vi "Heat fuse RV1.vi"(8 "error in":errorcluster) -> (0 "error out":errorcluster, 1 "PASS/FAIL":bool, 2 "VHeatFuse_load":string, 3 "VHeatFuse_noload":string)   [LabVIEW 2009]
uses:
  Digit IO PCI 6503/Digit IO control.ctl
  Global/Global 1.vi
panel:
  out "status":bool
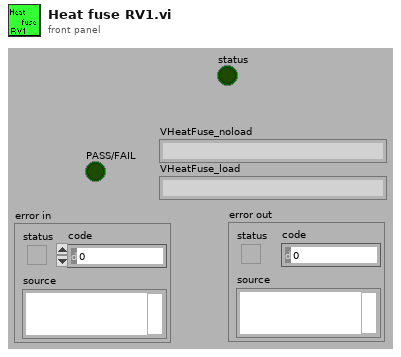
[diagram p1: front panel]
types:
  T1 = typedef "Digit IO control.ctl" = enum16{"Pull X1_4 Low", "Disconnect Pull X1_4 Low", "Down Cylinder", "Disconnect Down Cylinder", "Load X1_1_5", "Disconnect Load X1_1_5", "Measu X1_1_5", "Disconnect Measu X1_1_5", "Measu Z1_1_5", "Disconnect Measu Z1_1_5", "Power X1_1", "Disconnect Power X1_1", "RS232 Power", "Disconnect RS232 Power", "Card Cylinder", "Disconnect Card Cylinder", "Fail LED", "Disconnect Fail LED", "LCA Power", "Disconnect LCA Power", "BeyondCylinderDowndigit", "Disconnect BeyondCylinderDowendigit", "Frequency", "Disconnect Frequency", "Measu Current", "Disconnect Measu Current", "Measu current_1", "Disconnect Measu current_1", "Digit ALL", "Disconnect Digit ALL", "PASS LED", "Disconnect PASS LED", "Load Z1_1_3", "Disconnect Load Z1_1_3", "RS232 Connect", "Disconnect RS232 Connect", "Power Z1_7", "Disconnect Power Z1_7", "Pull Z_1_5  low", "Disconnect Pull Z_1_5  low", "Connect LCA_1", "Disconnect LCA_1", "short LCA", "Disconnect short LCA", "PT100", "Disconnect PT100", "NO connect", "Disconnect NO connect"}
  T2 = cluster{"VHEATFUSENOLOADMIN":string, "VHEATFUSELOADMAX":string, "VOVERRIDEDIODEMIN":string, "TDIFFMAX":string, "MEASFREQMAX":string, "MEASFREQMIN":string, "VOVER":string, "VMIDDLE":string, "VUNDER":string, "VNORESET":string, "VRESET":string, "WAITPING":string, "LRFID":string, "RFIDUID":string, "EXTEESIZE":string, "LCUTYPE":string, "LCUSUBTYPE":string, "TEVN":string, "BOOTVER":string, "APPVER":string, "ISLEEPMAX":string, "TSLEEP":string, "APPWAIT":string, "DBWAIT":string}
  T3 = cluster{"People":string, "product  number":string, "Test time":string, "VHeatFuse_noload":string, "VHeatFuse_load":string, "VoverrideDiode":string, "Test firmware upload via X1":string, "TemperAddress":string, "Troom":string, "TLCU":string, "Adjustment factor":string, "MeasuredFreq":string, "I2C communication":string, "Light-emitting diode on Z2":string, "Battery warning/inhibit":string, "Reset by IC10":string, "External EEPROM":string, "RFID card detection and reading RFID":string, "Production parameters in internal EEPROM":string, "Current consumption in sleep mode":string, "Application and database upload":string, "Test result":string, "Table head[22]":string, "Table head[23]":string}
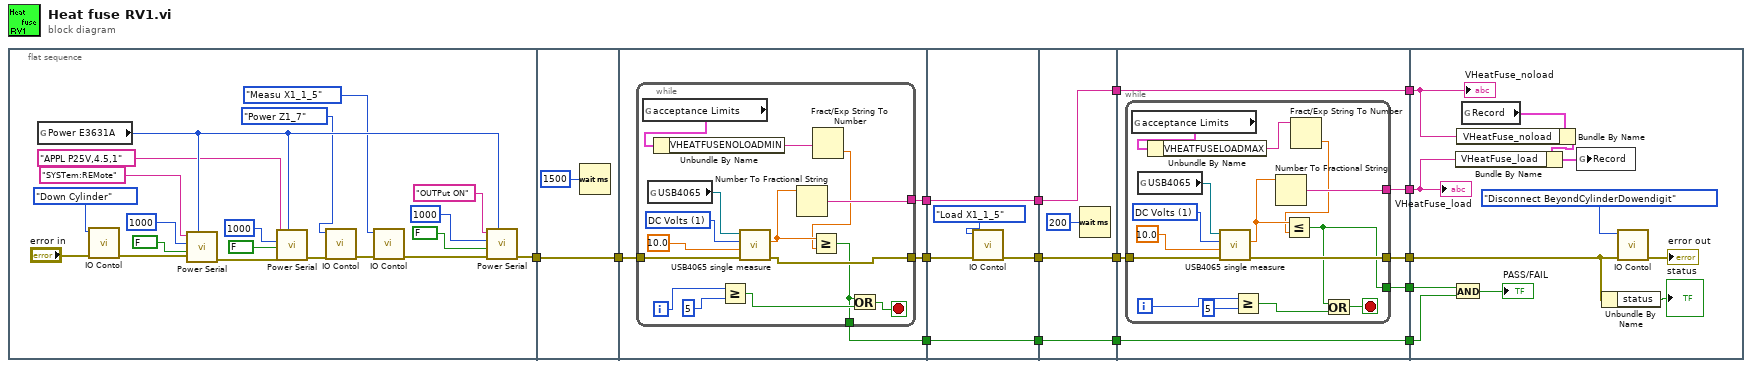
[diagram p0: block diagram]
diagram:
  n1 = flat-sequence {
    tunnel: [w33] -> w2
    tunnel: w2 -> [w37]
    tunnel: [w37] -> w1
    tunnel: [w42] -> w16
    tunnel: [w41] -> w8
    tunnel: [w40] -> w4
    tunnel: w1 -> [w39]
    tunnel: w16 -> [w62]
    tunnel: [w61] -> w14
    tunnel: [w59] -> w9
    tunnel: w8 -> [w59]
    tunnel: [w58] -> w5
    tunnel: w4 -> [w58]
    tunnel: [w65] -> w15
    tunnel: w14 -> [w65]
    tunnel: [w64] -> w10
    tunnel: w9 -> [w64]
    tunnel: [w63] -> w6
    tunnel: w5 -> [w63]
    tunnel: w15 -> [w72]
    tunnel: [w71] -> w13
    tunnel: [w70] -> w12
    tunnel: [w69] -> w11
    tunnel: w10 -> [w69]
    tunnel: [w68] -> w7
    tunnel: w6 -> [w68]
    tunnel: [w67] -> w3
    tunnel: w13 -> [w95]
    tunnel: w12 -> [w88]
    tunnel: w11 -> [w94]
    tunnel: w7 -> [w93]
    tunnel: w3 -> [w92]
    frame #0 {
      n2 = global read "Global 1.vi" "Power E3631A"() -> (w32:i32)
      n3 = call "IO Contol.vi"("error in"="error in", "IO Operation"=Digit_IO_control."Down Cylinder" ("Enum")) -> ("error out"=w17:errorcluster)  [unwired: 9 out]
      n4 = call "Power Serial.vi"("VISA Resource Address"=w32, "error in (no error)"=w17, "Rd?"=FALSE ("write"), "Delay"=1000, "IN"="SYSTem:REMote" ("In")) -> ("error out"=w24:errorcluster)  [unwired: 6 out]
      n5 = call "Power Serial.vi"("VISA Resource Address"=w32, "error in (no error)"=w24, "Rd?"=FALSE, "Delay"=1000, "IN"="APPL P25V,4.5,1" ("In")) -> ("error out"=w20:errorcluster)  [unwired: 6 out]
      n6 = call "IO Contol.vi"("error in"=w20, "IO Operation"=Digit_IO_control."Power Z1_7" ("Enum")) -> ("error out"=w30:errorcluster)  [unwired: 9 out]
      n7 = call "IO Contol.vi"("error in"=w30, "IO Operation"=Digit_IO_control."Measu X1_1_5" ("Enum")) -> ("error out"=w31:errorcluster)  [unwired: 9 out]
      n8 = call "Power Serial.vi"("VISA Resource Address"=w32, "error in (no error)"=w31, "Rd?"=FALSE, "Delay"=1000, "IN"="OUTPut ON" ("In")) -> ("error out"=w33:errorcluster)  [unwired: 6 out]
    }
    frame #1 {
      n9 = Wait (ms)(milliseconds to wait=u32 1500) -> ()  [unwired: 1 out]
    }
    frame #2 {
      n10 = while {
        tunnel: [w51] -> w42
        tunnel: [w45] -> w41
        tunnel: [w48] -> w40
        tunnel: w39 -> [w47]
        i -> [w54]
        stop <- w55 stop-if-true
        w57 = 1 items=["DC Volts"=1, "AC Volts"=2, "DC Current"=3, "AC Current"=4, "2-Wire Resistance"=5, "4-Wire Resistance"=101, "Frequency"=104, "Period"=105, "AC Volts DC Coupled"=1001, "Diode"=1002, "Waveform Voltage"=1003, "Waveform Current"=1004, "Capacitance"=1005, "Inductance"=1006, "Temperature"=108] ("Configuration:Function")
        n11 = global read "Global 1.vi" "acceptance Limits"() -> (w46:T2)
        n12 = global read "Global 1.vi" "USB4065"() -> (w50:refnum<k15>)
        n13 = Unbundle By Name(w46) -> ("VHEATFUSENOLOADMIN"=w44:string)
        n14 = Greater Or Equal?(x=w54, y=5) -> (x >= y?=w52:bool)
        n15 = call "USB4065 single measure.vi"("error in (no error)"=w47, "Configuration:Range"=10.0, "Configuration:Function"=w57, "Instrument Descriptor"=w50) -> ("error out"=w51:errorcluster, "Measurement"=w49:dbl)  [unwired: 6 out]
        n16 = Number To Fractional String(number=w49) -> (F-format string=w45:string)  [unwired: 3 out]
        n17 = Fract/Exp String To Number(string=w44) -> (number=w43:dbl)  [unwired: 4 out]
        n18 = Greater Or Equal?(x=w49, y=w43) -> (x >= y?=w48:bool)
        n19 = Or(x=w48, y=w52) -> (x .or. y?=w55:bool)
      }
    }
    frame #3 {
      n20 = call "IO Contol.vi"("error in"=w62, "IO Operation"=Digit_IO_control."Load X1_1_5" ("Enum")) -> ("error out"=w61:errorcluster)  [unwired: 9 out]
    }
    frame #4 {
      n21 = Wait (ms)(milliseconds to wait=u32 200) -> ()  [unwired: 1 out]
    }
    frame #5 {
      n22 = while {
        tunnel: w72 -> [w85]
        tunnel: [w75] -> w71
        tunnel: [w80] -> w70
        tunnel: [w77] -> w67
        i -> [w84]
        stop <- w82 stop-if-true
        w87 = 1 items=["DC Volts"=1, "AC Volts"=2, "DC Current"=3, "AC Current"=4, "2-Wire Resistance"=5, "4-Wire Resistance"=101, "Frequency"=104, "Period"=105, "AC Volts DC Coupled"=1001, "Diode"=1002, "Waveform Voltage"=1003, "Waveform Current"=1004, "Capacitance"=1005, "Inductance"=1006, "Temperature"=108] ("Configuration:Function")
        n23 = global read "Global 1.vi" "acceptance Limits"() -> (w76:T2)
        n24 = global read "Global 1.vi" "USB4065"() -> (w79:refnum<k15>)
        n25 = Unbundle By Name(w76) -> ("VHEATFUSELOADMAX"=w74:string)
        n26 = call "USB4065 single measure.vi"("error in (no error)"=w85, "Configuration:Range"=10.0, "Configuration:Function"=w87, "Instrument Descriptor"=w79) -> ("error out"=w80:errorcluster, "Measurement"=w78:dbl)  [unwired: 6 out]
        n27 = Greater Or Equal?(x=w84, y=5) -> (x >= y?=w81:bool)
        n28 = Number To Fractional String(number=w78) -> (F-format string=w75:string)  [unwired: 3 out]
        n29 = Fract/Exp String To Number(string=w74) -> (number=w73:dbl)  [unwired: 4 out]
        n30 = Less Or Equal?(x=w78, y=w73) -> (x <= y?=w77:bool)
        n31 = Or(x=w77, y=w81) -> (x .or. y?=w82:bool)
      }
    }
    frame #6 {
      n32 = And(x=w92, y=w93) -> (x .and. y?=→"PASS/FAIL":bool)
      n33 = global read "Global 1.vi" "Record"() -> (w98:T3)
      n34 = Bundle By Name(cluster=w98, "VHeatFuse_noload"=w94) -> (w97:T3)
      n35 = Bundle By Name(cluster=w97, "VHeatFuse_load"=w95) -> (w96:T3)
      n36 = global write "Global 1.vi" "Record"(w96) -> ()
      n37 = Unbundle By Name(w88) -> ("status"=→"status":bool)
      n38 = call "IO Contol.vi"("error in"=w88, "IO Operation"=Digit_IO_control."Disconnect BeyondCylinderDowendigit" ("Enum")) -> ("error out"=→"error out":errorcluster)  [unwired: 9 out]
      "VHeatFuse_load" <- w95
      "VHeatFuse_noload" <- w94
    }
  }
